vi "获取关键参数.vi"(8 "error in (no error)":errorcluster caption="错误输入（无错误）", 9 "量程":u16, 10 "flowid":u16, 11 "id":i32) -> (0 "error out":errorcluster caption="错误输出", 3 "关键参数":T1)   [LabVIEW 2016, in "斯坦道总磷总氮V2.lvlib"]
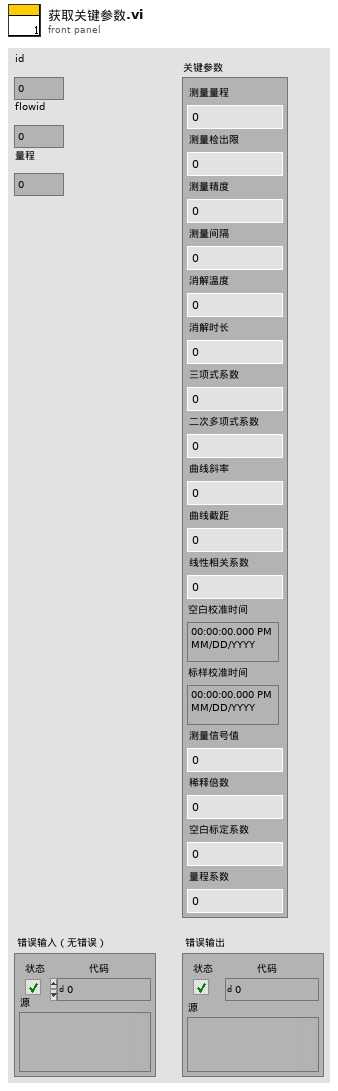
[diagram p1: front panel]
types:
  T1 = typedef "斯坦道总磷总氮V2.lvlib/关键参数.ctl" = cluster{"测量量程":sgl, "测量检出限":sgl, "测量精度":sgl, "测量间隔":sgl, "消解温度":sgl, "消解时长":sgl, "三项式系数":sgl, "二次多项式系数":sgl, "曲线斜率":sgl, "曲线截距":sgl, "线性相关系数":sgl, "空白校准时间":timestamp, "标样校准时间":timestamp, "测量信号值":sgl, "稀释倍数":sgl, "空白标定系数":sgl, "量程系数":sgl}
  T2 = cluster{"运行模式":enum16{"维护模式", "常规模式", "应急模式", "质控模式", "性能测试"}, "质控频次":enum16{"关闭", "每天", "星期一", "星期二", "星期三", "星期四", "星期五", "星期六", "星期日"}, "空白核查时间":u16, "跨度核查时间":u16, "测量间隔":dbl}
  T3 = cluster{"标液浓度1":dbl, "测量吸光度1":dbl, "样品1启用":bool, "标液浓度2":dbl, "测量吸光度2":dbl, "样品2启用":bool, "标液浓度3":dbl, "测量吸光度3":dbl, "样品3启用":bool, "标液浓度4":dbl, "测量吸光度4":dbl, "样品4启用":bool, "标液浓度5":dbl, "测量吸光度5":dbl, "样品5启用":bool, "模型":enum32{"线性", "多项式"}, "精度":dbl, "XY图":cluster{"X Values":dbl[], "Y Values":dbl[]}[], "拟合公式":string, "r^2":dbl, "标样一校准时间":timestamp, "标样二校准时间":timestamp, "标样三校准时间":timestamp, "标样四校准时间":timestamp, "标样五校准时间":timestamp, "二次方程":cluster{"c":dbl, "x":dbl, "x^2":dbl}, "标定时间":timestamp}
  T4 = cluster{"精度":dbl, "检出限":dbl, "量程上限":dbl, "量程下限":dbl}
  T5 = cluster{"标液浓度1":dbl, "测量吸光度1":dbl, "样品1启用":bool, "标液浓度2":dbl, "测量吸光度2":dbl, "样品2启用":bool, "标液浓度3":dbl, "测量吸光度3":dbl, "样品3启用":bool, "标液浓度4":dbl, "测量吸光度4":dbl, "样品4启用":bool, "标液浓度5":dbl, "测量吸光度5":dbl, "样品5启用":bool, "模型":enum32{"线性", "多项式"}, "精度":dbl, "XY图":cluster{"X Values":dbl[], "Y Values":dbl[]}[], "拟合公式":string, "r^2":dbl, "标样一校准时间":timestamp, "标样二校准时间":timestamp, "标样三校准时间":timestamp, "标样四校准时间":timestamp, "标样五校准时间":timestamp, "二次方程":cluster{"c":dbl, "x":dbl, "x^2":dbl}, "标定时间":timestamp}[]
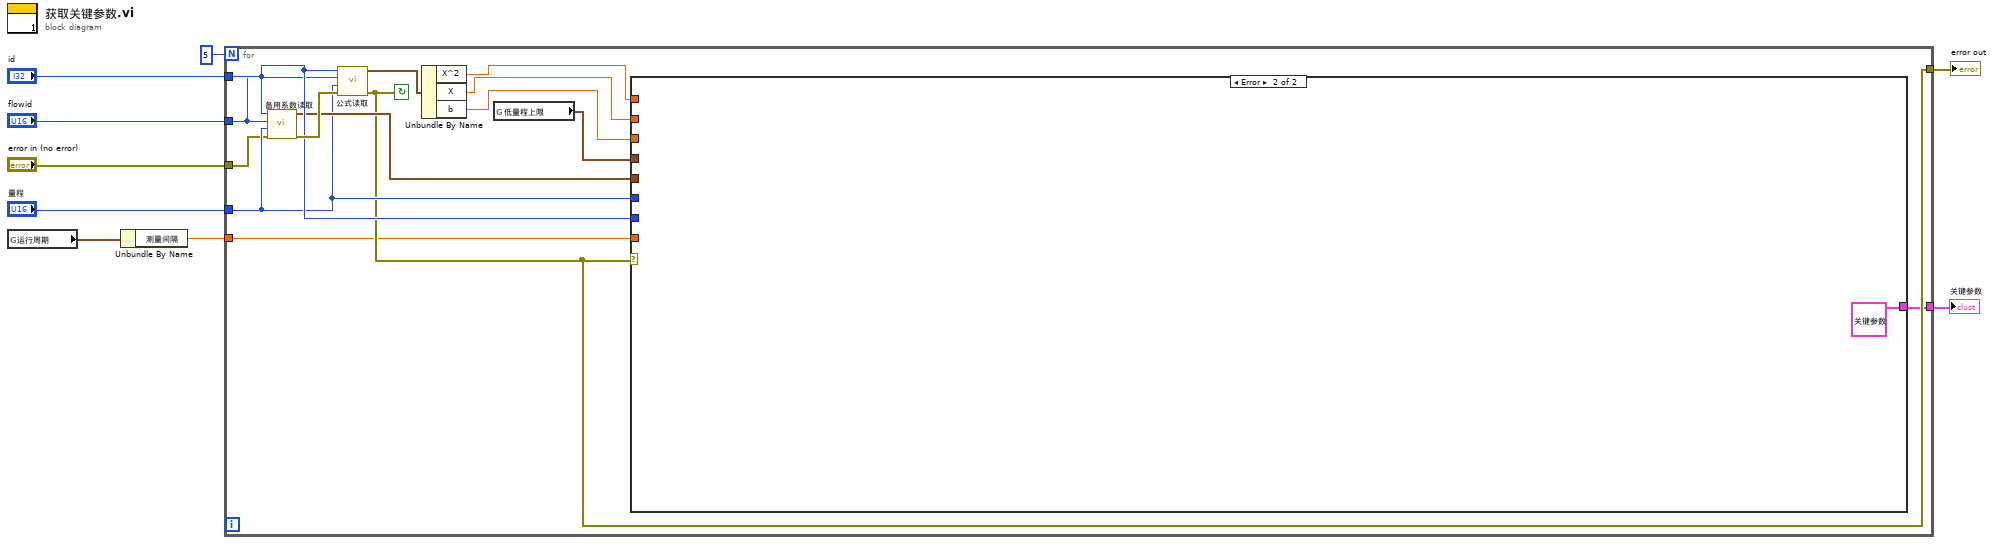
[diagram p0: block diagram]
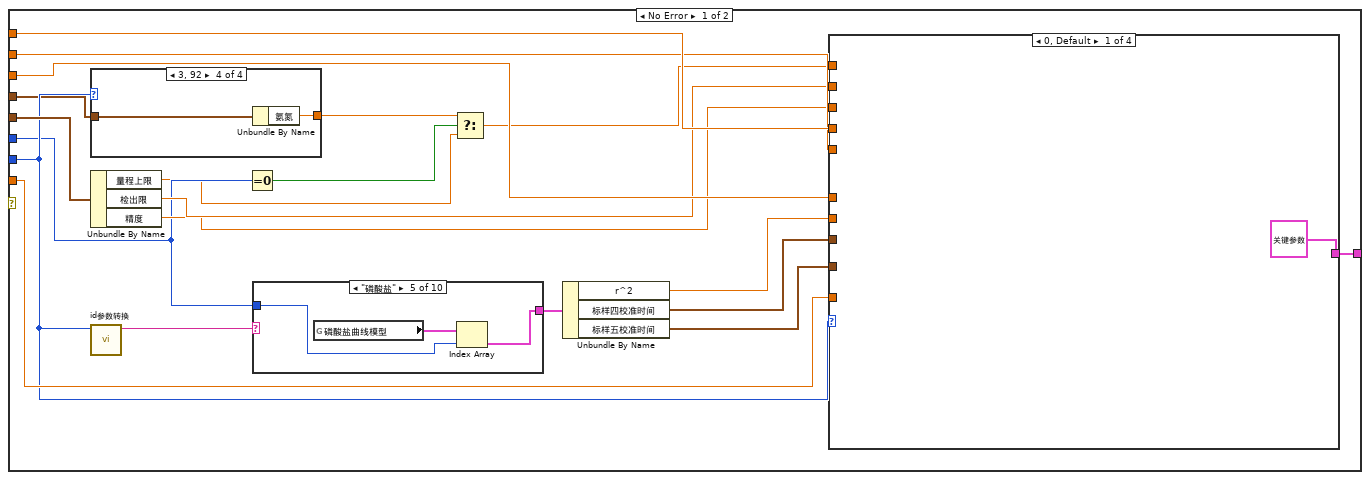
[diagram p2: hidden frame]
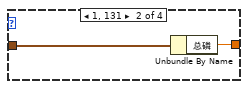
[diagram p4: hidden frame]
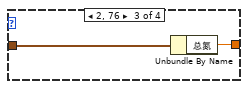
[diagram p5: hidden frame]
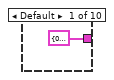
[diagram p6: hidden frame]
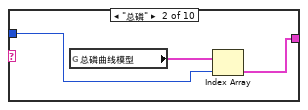
[diagram p7: hidden frame]
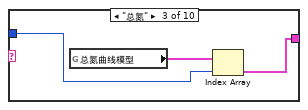
[diagram p8: hidden frame]
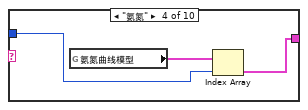
[diagram p9: hidden frame]
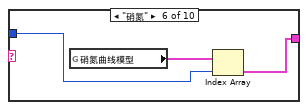
[diagram p10: hidden frame]
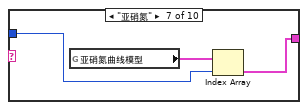
[diagram p11: hidden frame]
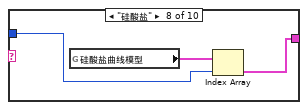
[diagram p12: hidden frame]
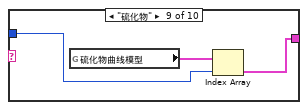
[diagram p13: hidden frame]
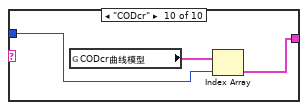
[diagram p14: hidden frame]
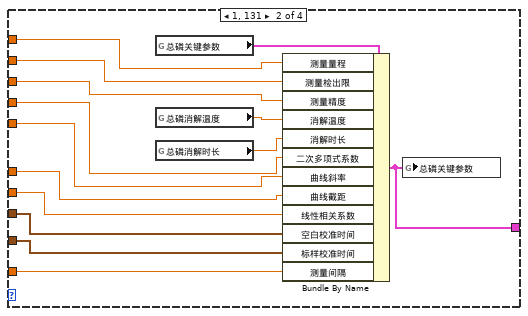
[diagram p15: hidden frame]
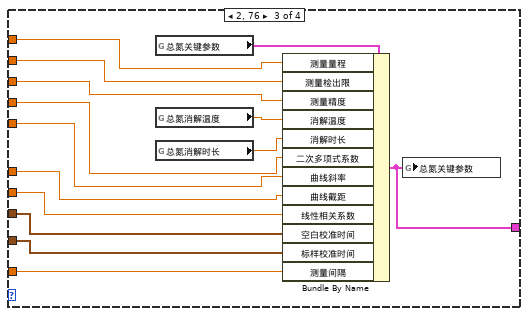
[diagram p16: hidden frame]
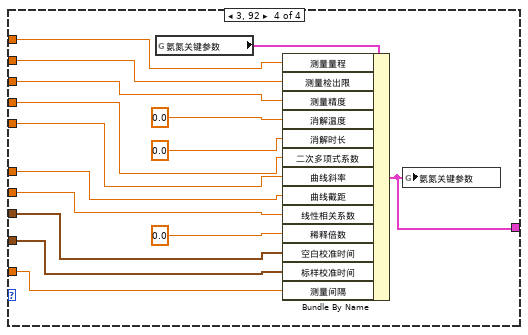
[diagram p17: hidden frame]
diagram:
  n1 = global read "总磷总氮断电保存全局变量.vi" "运行周期"() -> (w3:T2)
  n2 = Unbundle By Name(w3) -> ("测量间隔"=w2:dbl)
  n3 = for {
    N: 5 -> [_]
    tunnel: "量程" -> [w16]
    tunnel: "flowid" -> [w15]
    tunnel: "id" -> [w18]
    tunnel: "error in (no error)" -> [w14]
    tunnel: [w13] -> w4
    tunnel: w2 -> [w12]
    tunnel: [w10] -> w1
    stop <- w13 continue-if-true
    n4 = call "备用系数读取.vi"("error in (no error)"=w14, "量程下拉列表"=w16, "测量模式"=w15, "参数下拉列表"=w18) -> ("error out"=w19:errorcluster, "备用系数"=w17:T4)  [unwired: 6 in]
    n5 = call "公式读取.vi"("error in (no error)"=w19, "量程下拉列表"=w16, "测量模式"=w15, "参数下拉列表"=w18) -> ("error out"=w13:errorcluster, "公式"=w23:cluster{"X^2":dbl, "X":dbl, "b":dbl})  [unwired: 6 in]
    n6 = Unbundle By Name(w23) -> ("X^2"=w22:dbl, "X"=w21:dbl, "b"=w20:dbl)
    n7 = global read "总磷总氮断电保存全局变量.vi" "低量程上限"() -> (w11:cluster{"总磷":dbl, "总氮":dbl, "氨氮":dbl})
    n8 = case shown="Error" w13 {
      tunnel: w22 -> [w43 _]
      tunnel: w21 -> [w42 _]
      tunnel: w20 -> [w41 _]
      tunnel: w18 -> [w31 _]
      tunnel: w16 -> [w29 _]
      tunnel: w17 -> [w35 _]
      tunnel: w12 -> [w32 _]
      tunnel: w11 -> [w30 _]
      tunnel: [w24 T1 {"测量量程"=0.0, "测量检出限"=0.0, "测量精度"=0.0, "测量间隔"=0.0, "消解温度"=0.0, "消解时长"=0.0, "三项式系数"=0.0, "二次多项式系数"=0.0, "曲线斜率"=0.0, "曲线截距"=0.0, "线性相关系数"=0.0, "空白校准时间"=timestamp(0 s since 1904-01-01), "标样校准时间"=timestamp(0 s since 1904-01-01), "测量信号值"=0.0, "稀释倍数"=0.0, "空白标定系数"=0.0, "量程系数"=0.0} ("氨氮关键参数")] -> w10
      frame No Error {
        n9 = case shown="3, 92" w31 {
          tunnel: w30 -> [_ w45 w47 w49]
          tunnel: [_ w44 w46 w48] -> w27
          frame 0, Default {
          }
          frame 1, 131 {
            n10 = Unbundle By Name(w45) -> ("总磷"=w44:dbl)
          }
          frame 2, 76 {
            n11 = Unbundle By Name(w47) -> ("总氮"=w46:dbl)
          }
          frame 3, 92 {
            n12 = Unbundle By Name(w49) -> ("氨氮"=w48:dbl)
          }
        }
        n13 = Unbundle By Name(w35) -> ("量程上限"=w26:dbl, "检出限"=w34:dbl, "精度"=w33:dbl)
        n14 = call "id参数转换.vi"("id"=w31) -> ("table输出"=w40:string)  [unwired: 9 in, 1 out]
        n15 = Equal To 0?(x=w29) -> (x = 0?=w28:bool)
        n16 = case shown="\"磷酸盐\"" w40 {
          tunnel: w29 -> [_ w51 w54 w57 w60 w63 w66 w69 w72 w75]
          tunnel: [T3 {"标液浓度1"=0.0, "测量吸光度1"=0.0, "样品1启用"=FALSE, "标液浓度2"=0.0, "测量吸光度2"=0.0, "样品2启用"=FALSE, "标液浓度3"=0.0, "测量吸光度3"=0.0, "样品3启用"=FALSE, "标液浓度4"=0.0, "测量吸光度4"=0.0, "样品4启用"=FALSE, "标液浓度5"=0.0, "测量吸光度5"=0.0, "样品5启用"=FALSE, "模型"=enum."线性", "精度"=0.0, "XY图"=[], "拟合公式"="", "r^2"=0.0, "标样一校准时间"=timestamp(0 s since 1904-01-01), "标样二校准时间"=timestamp(0 s since 1904-01-01), "标样三校准时间"=timestamp(0 s since 1904-01-01), "标样四校准时间"=timestamp(0 s since 1904-01-01), "标样五校准时间"=timestamp(0 s since 1904-01-01), "二次方程"={"c"=0.0, "x"=0.0, "x^2"=0.0}, "标定时间"=timestamp(0 s since 1904-01-01)} ("总磷曲线模型") w52 w55 w58 w61 w64 w67 w70 w73 w76] -> w39
          frame Default {
          }
          frame "总磷" {
            n17 = global read "校准数据全局变量.vi" "总磷曲线模型"() -> (w53:T5)
            n18 = Index Array(array=w53, index=w51) -> (element=w52:T3)
          }
          frame "总氮" {
            n19 = global read "校准数据全局变量.vi" "总氮曲线模型"() -> (w56:T5)
            n20 = Index Array(array=w56, index=w54) -> (element=w55:T3)
          }
          frame "氨氮" {
            n21 = global read "校准数据全局变量.vi" "氨氮曲线模型"() -> (w59:T5)
            n22 = Index Array(array=w59, index=w57) -> (element=w58:T3)
          }
          frame "磷酸盐" {
            n23 = global read "校准数据全局变量.vi" "磷酸盐曲线模型"() -> (w62:T5)
            n24 = Index Array(array=w62, index=w60) -> (element=w61:T3)
          }
          frame "硝氮" {
            n25 = global read "校准数据全局变量.vi" "硝氮曲线模型"() -> (w65:T5)
            n26 = Index Array(array=w65, index=w63) -> (element=w64:T3)
          }
          frame "亚硝氮" {
            n27 = global read "校准数据全局变量.vi" "亚硝氮曲线模型"() -> (w68:T5)
            n28 = Index Array(array=w68, index=w66) -> (element=w67:T3)
          }
          frame "硅酸盐" {
            n29 = global read "校准数据全局变量.vi" "硅酸盐曲线模型"() -> (w71:T5)
            n30 = Index Array(array=w71, index=w69) -> (element=w70:T3)
          }
          frame "硫化物" {
            n31 = global read "校准数据全局变量.vi" "硫化物曲线模型"() -> (w74:T5)
            n32 = Index Array(array=w74, index=w72) -> (element=w73:T3)
          }
          frame "CODcr" {
            n33 = global read "校准数据全局变量.vi" "CODcr曲线模型"() -> (w77:T5)
            n34 = Index Array(array=w77, index=w75) -> (element=w76:T3)
          }
        }
        n35 = Select(t=w27, s=w28, f=w26) -> (s? t:f=w25:dbl)
        n36 = Unbundle By Name(w39) -> ("r^2"=w38:dbl, "标样四校准时间"=w37:timestamp, "标样五校准时间"=w36:timestamp)
        n37 = case shown="0, Default" w31 {
          tunnel: w43 -> [_ w90 w104 w120]
          tunnel: w42 -> [_ w89 w103 w119]
          tunnel: w41 -> [_ w88 w102 w118]
          tunnel: w38 -> [_ w85 w101 w115]
          tunnel: w37 -> [_ w86 w100 w114]
          tunnel: w36 -> [_ w87 w99 w113]
          tunnel: w25 -> [_ w83 w98 w111]
          tunnel: w34 -> [_ w82 w97 w110]
          tunnel: w33 -> [_ w81 w96 w109]
          tunnel: w32 -> [_ w80 w94 w108]
          tunnel: [T1 {"测量量程"=0.0, "测量检出限"=0.0, "测量精度"=0.0, "测量间隔"=0.0, "消解温度"=0.0, "消解时长"=0.0, "三项式系数"=0.0, "二次多项式系数"=0.0, "曲线斜率"=0.0, "曲线截距"=0.0, "线性相关系数"=0.0, "空白校准时间"=timestamp(0 s since 1904-01-01), "标样校准时间"=timestamp(0 s since 1904-01-01), "测量信号值"=0.0, "稀释倍数"=0.0, "空白标定系数"=0.0, "量程系数"=0.0} ("氨氮关键参数") w79 w93 w107] -> w24
          frame 0, Default {
          }
          frame 1, 131 {
            n38 = global read "VAR总磷总氮全局变量.vi" "总磷关键参数"() -> (w92:T1)
            n39 = global read "总磷总氮断电保存全局变量.vi" "总磷消解温度"() -> (w84:dbl)
            n40 = global read "总磷总氮断电保存全局变量.vi" "总磷消解时长"() -> (w91:dbl)
            n41 = Bundle By Name(cluster=w92, "测量量程"=w83, "测量检出限"=w82, "测量精度"=w81, "消解温度"=w84, "消解时长"=w91, "二次多项式系数"=w90, "曲线斜率"=w89, "曲线截距"=w88, "线性相关系数"=w85, "空白校准时间"=w86, "标样校准时间"=w87, "测量间隔"=w80) -> (w79:T1)
            n42 = global write "VAR总磷总氮全局变量.vi" "总磷关键参数"(w79) -> ()
          }
          frame 2, 76 {
            n43 = global read "VAR总磷总氮全局变量.vi" "总氮关键参数"() -> (w106:T1)
            n44 = global read "总磷总氮断电保存全局变量.vi" "总氮消解温度"() -> (w95:dbl)
            n45 = global read "总磷总氮断电保存全局变量.vi" "总氮消解时长"() -> (w105:dbl)
            n46 = Bundle By Name(cluster=w106, "测量量程"=w98, "测量检出限"=w97, "测量精度"=w96, "消解温度"=w95, "消解时长"=w105, "二次多项式系数"=w104, "曲线斜率"=w103, "曲线截距"=w102, "线性相关系数"=w101, "空白校准时间"=w100, "标样校准时间"=w99, "测量间隔"=w94) -> (w93:T1)
            n47 = global write "VAR总磷总氮全局变量.vi" "总氮关键参数"(w93) -> ()
          }
          frame 3, 92 {
            n48 = global read "VAR总磷总氮全局变量.vi" "氨氮关键参数"() -> (w121:T1)
            n49 = Bundle By Name(cluster=w121, "测量量程"=w111, "测量检出限"=w110, "测量精度"=w109, "消解温度"=sgl 0.0, "消解时长"=sgl 0.0, "二次多项式系数"=w120, "曲线斜率"=w119, "曲线截距"=w118, "线性相关系数"=w115, "稀释倍数"=sgl 0.0, "空白校准时间"=w114, "标样校准时间"=w113, "测量间隔"=w108) -> (w107:T1)
            n50 = global write "VAR总磷总氮全局变量.vi" "氨氮关键参数"(w107) -> ()
          }
        }
      }
      frame Error {
      }
    }
  }
  "error out" <- w4
  "关键参数" <- w1
